vi "RealNumberCompare.vi"(1 "Percent? (Default F)":bool, 2 "Difference?":dbl=0.001, 3 "Number 2":dbl, 4 "Number 1":dbl) -> (0 "Equal to?":bool)   [LabVIEW 2012]
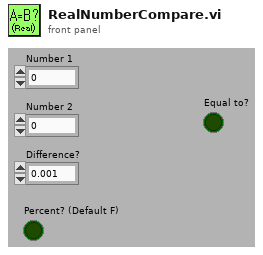
[diagram p1: front panel]
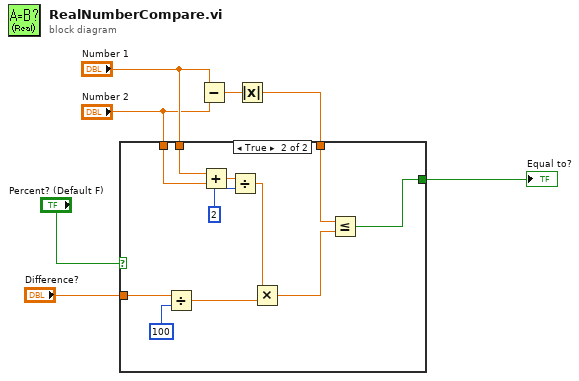
[diagram p0: block diagram]
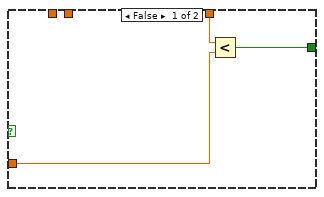
[diagram p2: hidden frame]
diagram:
  n1 = Subtract(x="Number 1", y="Number 2") -> (x-y=w7:dbl)
  n2 = Absolute Value(x=w7) -> (abs(x)=w6:dbl)
  n3 = case shown="True" "Percent? (Default F)" {
    tunnel: w6 -> [w10 w15]
    tunnel: [w9 w13] -> w5
    tunnel: "Number 1" -> [_ w21]
    tunnel: "Number 2" -> [_ w20]
    tunnel: "Difference?" -> [w8 w17]
    frame False {
      n4 = Less?(x=w10, y=w8) -> (x < y?=w9:bool)
    }
    frame True {
      n5 = Divide(x=w17, y=100) -> (x/y=w12:dbl)
      n6 = Add(x=w21, y=w20) -> (x+y=w19:dbl)
      n7 = Divide(x=w19, y=2) -> (x/y=w16:dbl)
      n8 = Multiply(x=w16, y=w12) -> (x*y=w14:dbl)
      n9 = Less Or Equal?(x=w15, y=w14) -> (x <= y?=w13:bool)
    }
  }
  "Equal to?" <- w5
